vi "调整角度.vi"(8 "调整":dbl, 11 "原角度":dbl) -> (2 "调整后 角度值":dbl)   [LabVIEW 2016]
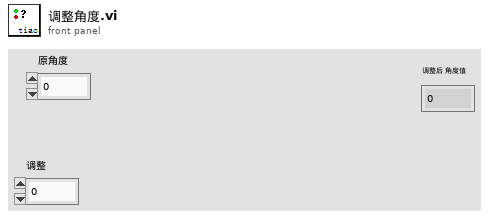
[diagram p1: front panel]
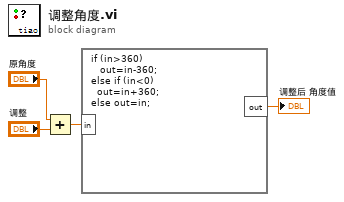
[diagram p0: block diagram]
diagram:
  n1 = Add(x="原角度", y="调整") -> (x+y=w3:dbl)
  n2 = formula code="if (in>360)\n   out=in-360;\nelse if (in<0)\n  out=in+360;\nelse out=in;"("in"=w3) -> ("out"=→"调整后 角度值":dbl)
